vi "Kinect Demo.vi"() -> ()   [LabVIEW 2011]
panel:
  out "Depth Image":T1(plugin-control)
  in  "stop":bool
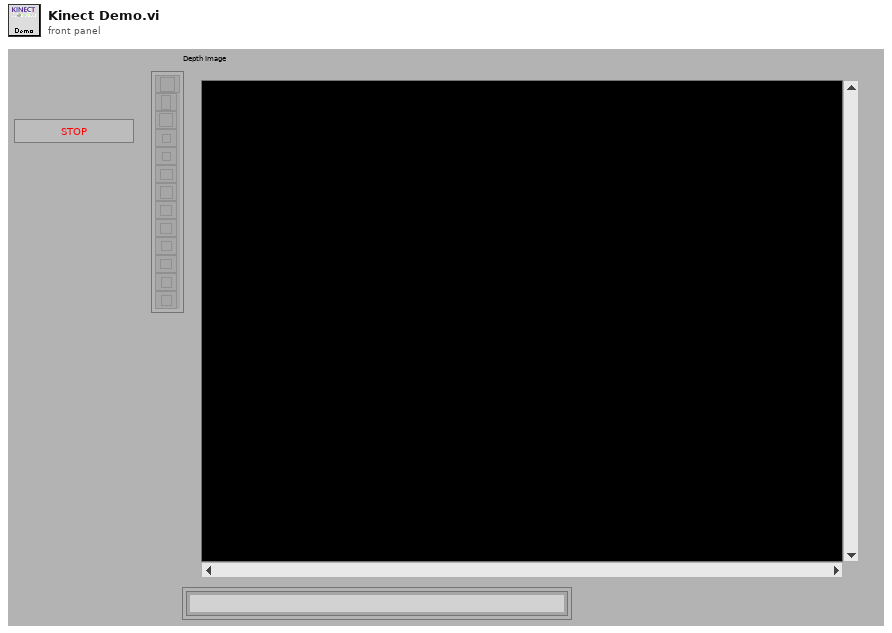
[diagram p1: front panel]
types:
  T1 = typedef "IMAQ Image.ctl" = refnum<image>
  T2 = cluster{cluster{"queue out":refnum<queue>}, cluster{"get_Item":refnum<k24>, "DepthStream":refnum<k24>, "Event Callback":refnum<k27>}}
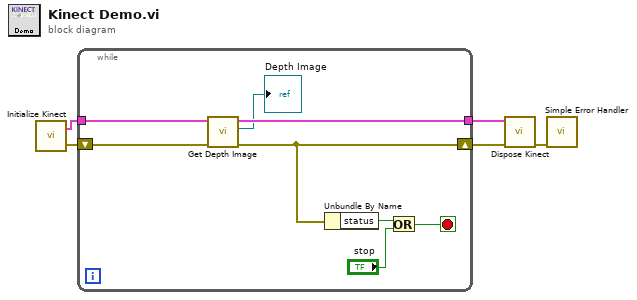
[diagram p0: block diagram]
diagram:
  n1 = call "Initialize Kinect.vi"() -> ("output cluster"=w5:T2, "Error Out"=w4:errorcluster)  [unwired: 1 in]
  n2 = while {
    shift-right: [w7] -> w3
    shift-left: w4 -> [w8]
    tunnel: w5 -> [w10]
    tunnel: [w9] -> w1
    stop <- w11 stop-if-true
    n3 = call "Get Depth Image.vi"("error in (no error)"=w8, "in cluster"=w10) -> ("error out"=w7:errorcluster, "Depth Image"=→"Depth Image":T1, "out cluster"=w9:T2)  [unwired: 4 in, 1 out]
    n4 = Unbundle By Name(w7) -> ("status"=w13:bool)
    n5 = Or(x=w13, y="stop") -> (x .or. y?=w11:bool)
  }
  n6 = call "Dispose Kinect.vi"("error in (no error)"=w3, "input cluster"=w1) -> ("error out"=w2:errorcluster)  [unwired: 9 in]
  n7 = call <vilib>:"Simple Error Handler.vi"("error in (no error)"=w2) -> ()  [unwired: 4 in, 5 out]
